vi "Control_Channel_Status.vi"() -> ()   [LabVIEW 2016]
uses:
  Sub VIs/ADAM Controls/Channel_State.ctl
  Sub VIs/ADAM Controls/Channel_names.ctl
  Anemometry/Anemometry Sub Vis/Globals/Preference_global.vi
panel:
  out "List of Addresses":string[](array[string])
  in  "Address":u16(ring) items=["Show All", "0", "161", "162", "164", "168", "169", "170", "174", "175", "502"]
  out "List of Ports":string[](array[string])
  in  "Port Names":u16(ring) items=["Show All", "", "CSUWebClient.vi", "CFWSWebClient.vi", "CSPressureSelector.vi", "192.168.124.56", "192.168.126.156", "tcp://192.168.126.152:10001/", "192.168.126.155"]
  out "Turn On?":bool
  in  "Turn Channel Off?":bool
  in  "stop":bool
  out "Ch State":T1
  in  "Turn Channels On?":bool
  in  "Selected Channels to Edit":i32[](listbox)
  in  "Search Charcters":string
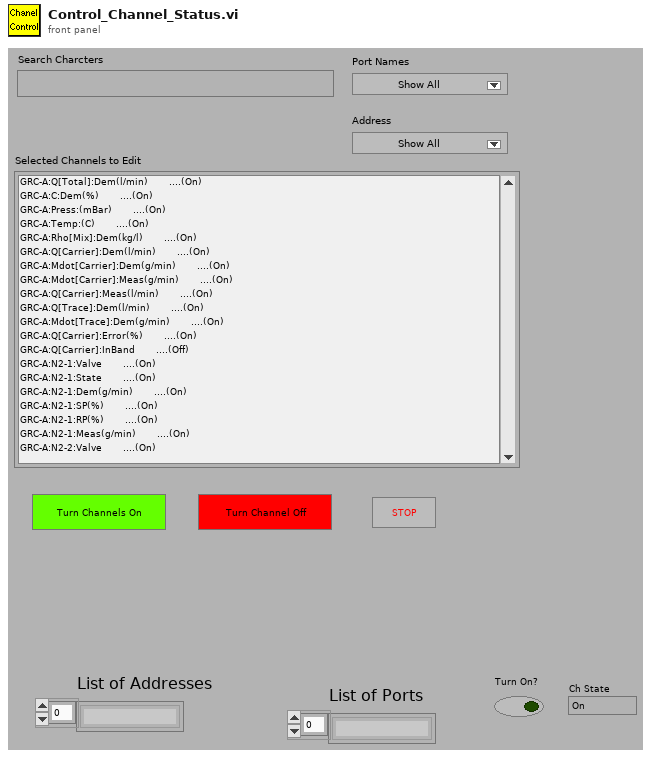
[diagram p1: front panel]
types:
  T1 = typedef "Channel_State.ctl" = enum16{"On", "Off", "Always On", "Always Off"}
  T2 = typedef "Channel_names.ctl" = enum16{"Active Only", "Active + Off", "All Channels"}
  T3 = typedef "Server_Comms.ctl" = enum16{"Server Link Healthy", "Do Not Link To Server"}
  T4 = typedef "Ch_description_ADAM.ctl" = cluster{"Ch Name":string, "Type":T5, "Function":T6, "Ch State":T1, "Calibration type":T7, "A":dbl, "B":dbl, "C":dbl, "D":dbl, "Comments":string, "Address":T8, "String":string, "Duty":u16}
  T5 = typedef "Module_type_ADAM.ctl" = string
  T6 = typedef "Function_ADAM.ctl" = enum16{"Analogue Input", "Digital Input", "Event counter", "Event rate", "Analogue Output", "Digital Output", "Relay Output"}
  T7 = typedef "Calib_type_ADAM.ctl" = string
  T8 = typedef "Address.ctl" = cluster{"Main":i32, "Ch.":i32, "Sub":i32, "Port Name":string}
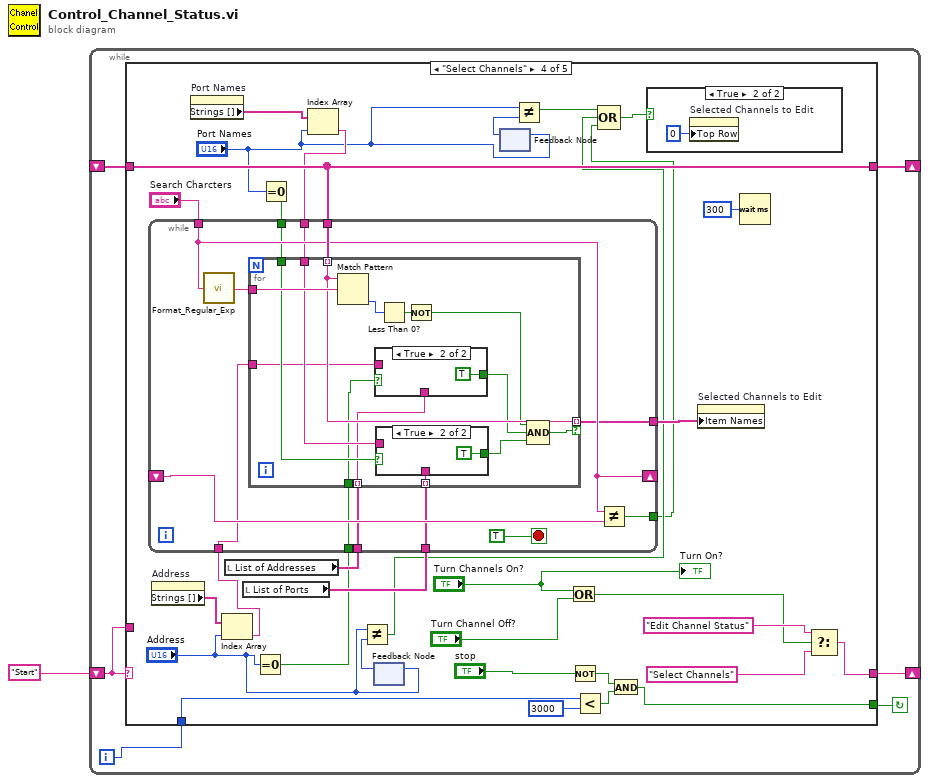
[diagram p0: block diagram]
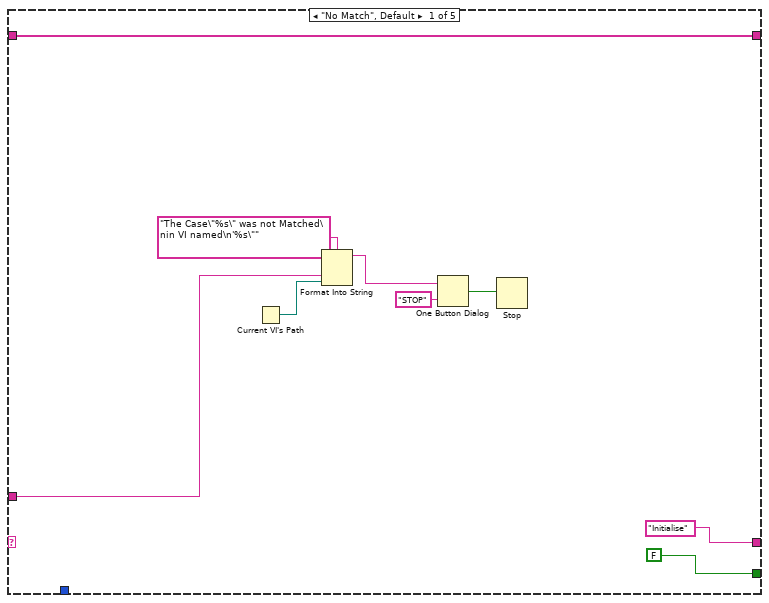
[diagram p2: hidden frame]
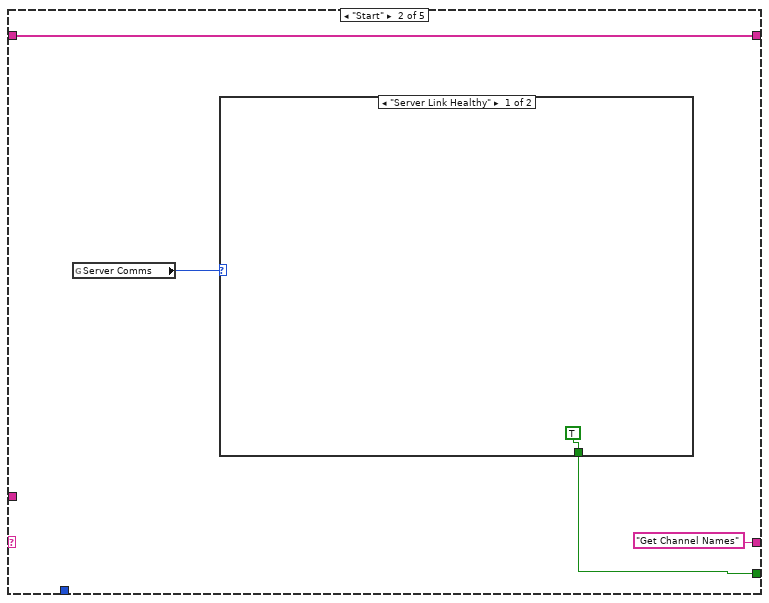
[diagram p3: hidden frame]
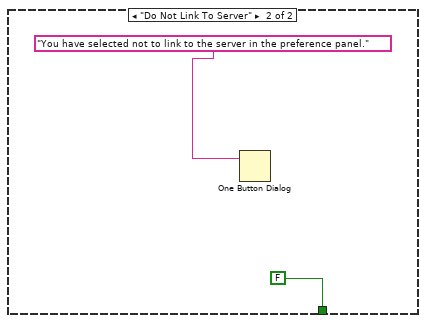
[diagram p4: hidden frame]
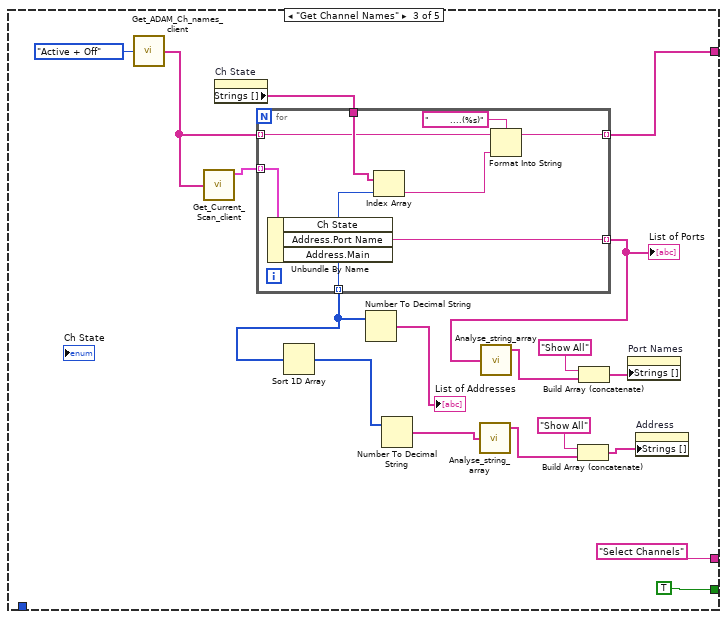
[diagram p5: hidden frame]
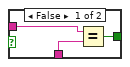
[diagram p7: hidden frame]
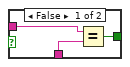
[diagram p8: hidden frame]
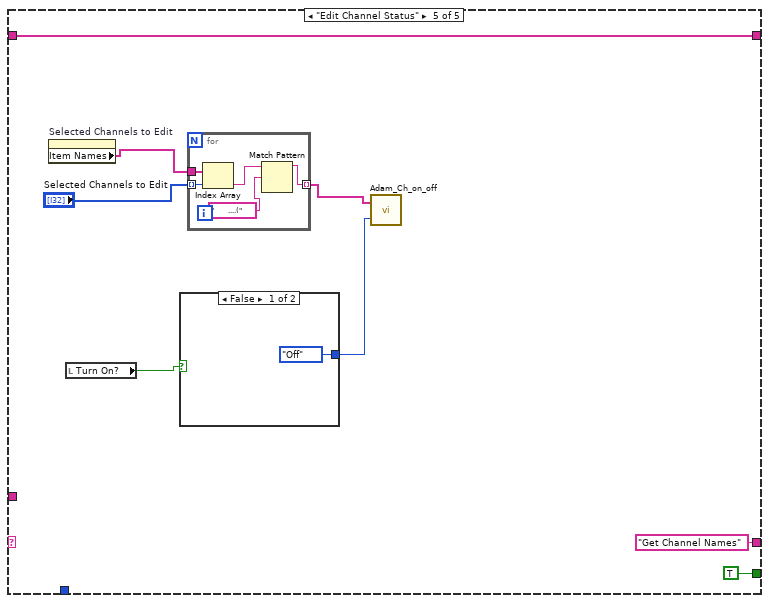
[diagram p9: hidden frame]
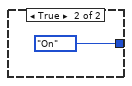
[diagram p10: hidden frame]
diagram:
  n1 = while {
    shift-left: "Start" -> [w5]
    shift-right: [w6] -> _
    shift-right: [w4] -> _
    shift-left: _ -> [w3]
    i -> [w2]
    stop <- w7 continue-if-true
    n2 = case shown="\"Select Channels\"" w5 {
      tunnel: [FALSE w18 TRUE w69 TRUE] -> w7
      tunnel: ["Initialise" "Get Channel Names" "Select Channels" w79 "Get Channel Names"] -> w6
      tunnel: w5 -> [w11 _ _ _ _]
      tunnel: [w8 w17 w35 w77 w126] -> w4
      tunnel: w3 -> [w8 w17 _ w77 w126]
      tunnel: w2 -> [_ _ _ w68 _]
      frame "No Match", Default {
        n3 = Current VI's Path() -> (path=w10:path)
        n4 = Format Into String(format string="The Case\"%s\" was not Matched\nin VI named\n'%s\"" ("Format String"), w11, w10) -> (resulting string=w14:string)  [unwired: 2 in, 1 out]
        n5 = One Button Dialog(message=w14, button name ("OK")="STOP") -> (true=w12:bool)
        n6 = Stop(stop? (T)=w12) -> ()
      }
      frame "Start" {
        n7 = global read "Preference_global.vi" "Server Comms"() -> (w19:T3)
        n8 = case shown="\"Server Link Healthy\"" w19 {
          tunnel: [TRUE FALSE] -> w18
          frame "Server Link Healthy" {
          }
          frame "Do Not Link To Server" {
            n9 = One Button Dialog(message="You have selected not to link to the server in the preference panel.") -> ()  [unwired: 2 out]
          }
        }
      }
      frame "Get Channel Names" {
        n10 = call "Get_ADAM_Ch_names_client.vi"("Channel names set"=Channel_names."Active + Off") -> ("Ch names"=w36:string[])
        n11 = call "Get_Current_Scan_client.vi"("ADAM Ch Names"=w36) -> ("Ch Description Array"=w38:T4[])  [unwired: 3 out]
        n12 = property on="Ch State" class="Enum (strict)"() -> ("Strings []"=w37:string[])  [unwired: 2 in, 2 out]
        n13 = for {
          tunnel: w38 -> [w50] mode=indexing
          tunnel: w37 -> [w49]
          tunnel: w36 -> [w47] mode=indexing
          tunnel: [w44] -> w35 mode=indexing
          tunnel: [w43] -> w34 mode=indexing
          tunnel: [w42] -> w25 mode=indexing
          n14 = Unbundle By Name(w50) -> ("Ch State"=w48:T1, "Address.Port Name"=w43:string, "Address.Main"=w42:i32)
          n15 = Index Array(array=w49, index=w48) -> (element=w46:string)
          n16 = Format Into String(format string="       ....(%s)", initial string=w47, w46) -> (resulting string=w44:string)  [unwired: 1 in, 1 out]
        }
        "List of Ports" <- w34
        n17 = Sort 1D Array(array=w25) -> (sorted array=w27:i32[])
        n18 = Number To Decimal String(number=w25) -> (decimal integer string=→"List of Addresses":string[])  [unwired: 1 in]
        n19 = Number To Decimal String(number=w27) -> (decimal integer string=w26:string[])  [unwired: 1 in]
        n20 = call "Analyse_string_array.vi"("String array"=w26) -> ("Unique strings"=w29:string[])  [unwired: 1 in, 1 out]
        n21 = call "Analyse_string_array.vi"("String array"=w34) -> ("Unique strings"=w33:string[])  [unwired: 1 in, 1 out]
        n22 = Build Array (concatenate)("Show All", w29) -> (w28:string[])
        n23 = Build Array (concatenate)("Show All", w33) -> (w31:string[])
        n24 = property on="Port Names" class="Ring (strict)"("Strings []"=w31) -> ()  [unwired: 2 in, 2 out]
        n25 = property on="Address" class="Ring (strict)"("Strings []"=w28) -> ()  [unwired: 2 in, 2 out]
      }
      frame "Select Channels" {
        n26 = property on="Address" class="Ring (strict)"() -> ("Strings []"=w61:string[])  [unwired: 2 in, 2 out]
        n27 = property on="Port Names" class="Ring (strict)"() -> ("Strings []"=w66:string[])  [unwired: 2 in, 2 out]
        n28 = Index Array(array=w61, index="Address") -> (element=w58:string)
        n29 = local read "List of Addresses"() -> (w59:string[])
        n30 = local read "List of Ports"() -> (w60:string[])
        n31 = Equal To 0?(x="Address") -> (x = 0?=w57:bool)
        n32 = Equal To 0?(x="Port Names") -> (x = 0?=w64:bool)
        n33 = Index Array(array=w66, index="Port Names") -> (element=w65:string)
        n34 = while {
          tunnel: [w90] -> w82
          tunnel: w77 -> [w96]
          tunnel: "Search Charcters" -> [w94]
          shift-right: [w94] -> _
          shift-left: _ -> [w93]
          tunnel: [w92] -> w51
          tunnel: w65 -> [w89]
          tunnel: w64 -> [w88]
          tunnel: w60 -> [w87]
          tunnel: w59 -> [w86]
          tunnel: w58 -> [w85]
          tunnel: w57 -> [w84]
          stop <- TRUE stop-if-true
          n35 = call "Format_Regular_Exp.vi"("Regular expression"=w94) -> ("Case Insensitive for html"=w95:string)
          n36 = for {
            tunnel: w95 -> [w110]
            tunnel: w96 -> [w108] mode=indexing
            tunnel: [w108] -> w90 mode=indexing if=w103
            tunnel: w89 -> [w105]
            tunnel: w87 -> [w106] mode=indexing
            tunnel: w88 -> [w102]
            tunnel: w86 -> [w101] mode=indexing
            tunnel: w85 -> [w100]
            tunnel: w84 -> [w99]
            n37 = Match Pattern(string=w108, regular expression=w110) -> (offset past match=w109:i32)  [unwired: 4 out]
            n38 = case shown="True" w99 {
              tunnel: w101 -> [w113 _]
              tunnel: w100 -> [w112 _]
              tunnel: [w111 TRUE] -> w97
              frame False {
                n39 = Equal?(x=w112, y=w113) -> (x = y?=w111:bool)
              }
              frame True {
              }
            }
            n40 = case shown="True" w102 {
              tunnel: w106 -> [w117 _]
              tunnel: w105 -> [w116 _]
              tunnel: [w115 TRUE] -> w104
              frame False {
                n41 = Equal?(x=w116, y=w117) -> (x = y?=w115:bool)
              }
              frame True {
              }
            }
            n42 = Less Than 0?(x=w109) -> (x < 0?=w107:bool)
            n43 = Not(x=w107) -> (.not. x?=w98:bool)
            n44 = Compound Arithmetic op=AND(w98, w97, w104) -> (w103:bool)
          }
          n45 = Not Equal?(x=w94, y=w93) -> (x != y?=w92:bool)
        }
        n46 = feedback #1() -> (w56:u16)  [unwired: 1 in]
        n47 = Not Equal?(x="Address", y=w56) -> (x != y?=w53:bool)
        n48 = feedback-in #1("Address") -> ()
        n49 = feedback-in #2("Port Names") -> ()
        n50 = feedback #2() -> (w63:u16)  [unwired: 1 in]
        n51 = Not Equal?(x="Port Names", y=w63) -> (x != y?=w54:bool)
        n52 = Or(x="Turn Channels On?", y="Turn Channel Off?") -> (x .or. y?=w72:bool)
        n53 = Not(x="stop") -> (.not. x?=w71:bool)
        n54 = Less?(x=w68, y=3000) -> (x < y?=w70:bool)
        n55 = Compound Arithmetic op=OR(w54, w53, w51) -> (w52:bool)
        n56 = And(x=w71, y=w70) -> (x .and. y?=w69:bool)
        n57 = case shown="True" w52 {
          frame False {
          }
          frame True {
            n58 = property on="Selected Channels to Edit" class="LstBox (strict)"("Top Row"=0) -> ()  [unwired: 2 in, 2 out]
          }
        }
        n59 = property on="Selected Channels to Edit" class="LstBox (strict)"("Item Names"=w82) -> ()  [unwired: 2 in, 2 out]
        n60 = Wait (ms)(milliseconds to wait=u32 300) -> ()  [unwired: 1 out]
        n61 = Select(t="Edit Channel Status", s=w72, f="Select Channels") -> (s? t:f=w79:string)
        "Turn On?" <- "Turn Channels On?"
      }
      frame "Edit Channel Status" {
        n62 = property on="Selected Channels to Edit" class="LstBox (strict)"() -> ("Item Names"=w122:string[])  [unwired: 2 in, 2 out]
        n63 = local read "Turn On?"() -> (w120:bool)
        n64 = case shown="False" w120 {
          tunnel: [Channel_State."Off" ("Ch State") Channel_State."On" ("Ch State")] -> w119
          frame False {
          }
          frame True {
          }
        }
        n65 = for {
          tunnel: "Selected Channels to Edit" -> [w133] mode=indexing
          tunnel: w122 -> [w132]
          tunnel: [w131] -> w121 mode=indexing
          n66 = Index Array(array=w132, index=w133) -> (element=w129:string)
          n67 = Match Pattern(string=w129, regular expression="       ....(" ("format string")) -> (before substring=w131:string)  [unwired: 4 out]
        }
        n68 = call "Adam_Ch_on_off.vi"("Ch State"=w119, "ADAM Ch Names"=w121) -> ()  [unwired: 1 out]
      }
    }
  }
